vi "Save FITS with Headers coop.vi"(4 "FITS info":T1={"File name"="lsob_demo_0530_LM_20190529_124525_live_C1_00020_001_lev0.0.fits", "Date"="2019-05-29T12:45:25"}, 5 "Camera.lvclass":refnum<class "Camera.lvclass">, 6 "byte order (0:big-endian, network order)":T12(ring), 7 "SCD FITS Cluster":T2={"Wavelength (nm)"=530.15, "Exposure (s)"=0.05, "Tuning Delay (ms)"=1000.0, "Beam Type (-1/1)"=1.0, "Tuning Voltages"=[1.111, 2.222, 3.333, 4.444], "Observer"="observer", "Light Shapping Diffuser"=enum."In Beam", "Comment"="", "Data Type"=enum."HOLE", "Mod Cycles"=0, "SCD Calibration Optics"=enum."1 - Polarizer @0, I+Q", "SCD Emission Line Filter"=enum."1-557.6nm", "Cookbook"="", "COMP-S Calibration Wheel"=enum."Dark", "COMP-S Andover Filter Wheel"=enum."530.3nm/HWB 0.34nm (Fe XIV)", "FOV Rotation (deg)"=66.0, "Objective Lens Position (mm)"=0.0, "Occulter size"=0.0, "Time End"=timestamp(3382374145.421875 s since 1904-01-01), "Acc Exposure (s)"=0.0, "Time Stamp Array"=[], "Camera Serial Number"=[], "Camera Temp"=[], "Camera PI (mm)"=[], "Time Start"=timestamp(3382374145.421875 s since 1904-01-01), "Peripherals"={"ILX controler"=FALSE, "Zone temperatures"=FALSE, "Andor"=FALSE, "Andor 2"=FALSE, "PI Stages"=FALSE, "AISAS mechanisms"=FALSE, "AISAS Mech.lvclass"=refnum, "Zone temp ref"=variant, "FWs"=FALSE}, "FITS paths"=[], "Cameras"=enum."Andor", "load preset cbk"=FALSE, "periodic check count"=0, "COMP-S Calibration Wheel 2"=enum."Dark", "Calib"=enum."Dark", "Abso Aperture"=66.0, "Nominal Aperture"=66.0} {"Nominal Aperture" format="%.1f"; "Abso Aperture" format="%.1f"; "Camera PI (mm)" format="%_3g"; "Acc Exposure (s)" format="%^.3g"; "Occulter size" format="%.2f"; "Objective Lens Position (mm)" min=70.0 max=152.0 format="%.2f"; "FOV Rotation (deg)" format="%.1f"; "Exposure (s)" format="%^.3g"; "Wavelength (nm)" format="%_6g"}, 8 "error in":errorcluster, 9 "Image Data":u32[](array[numeric]), 10 "Image #":i32=1, 11 "FITS File Path":path=path "G:/SCD Data/Level-0/20160930/20160930T203514.fits") -> (0 "error out":errorcluster, 2 "23040 Byte Header":string="SIMPLE  =                              T / CONFORMS TO FITS STANDARD            BITPIX  =                             32 / BITS PER PIXEL                       NAXIS   =                              2 / DATA DIMENSIONS IN FITS FILE         NAXIS1  =                              0 / XDIM (PIXELS)                        NAXIS2  =                              0 / YDIM (PIXELS)                        NAXIS3  =                              4 / 4 POLARIZATION STATES                NAXIS4  =                              1 / 1 CAMERA                             ORIGIN  =                        'AISAS' / SCIENTIFIC GROUP                     OBSERVER=                     'SCHWARTZ' / NAME OF OBSERVER                     TELESCOP=                   '20CM ZEISS' / NAME OF TELESCOPE                    LOCATION=            'LOMNICKY PEAK OBS' / LOCATION OF TELESCOPE                INSTRUME=                          'SCD' / NAME OF INSTRUMENT                   BZERO   =                             0. /  ADU OFFSET                          FOCUS   =                             26 / CAMERA-STAGE POSITION (MM)           ROTPOS  =                           66.0 / ROTATIONAL POSITION (DEG)            DIFFUSER=                      'IN BEAM' / 0=IN BEAM, 1=OUT OF BEAM             FW-WVLNG=                        '557.6' / PRE-FILTER CENTER WAVELENGTH (NM)    FW-CALIB=                         'DARK' / CAL-WHEEL POSITION                   CAM-SN1 =                    'SCC-02209' / CAMERA SERIAL NUMBER                 CAM-TEMP=                       0.000000 / FOCAL PLANE TEMP (C)                 TUNEDLAY=                           1000 / LCVR RELAXATION DELAY (mS)           DATE_OBS=                     '3/7/2011' / DATE OF OBSERVATION START (UTC)      TIME_OBS=                   '212225.421' / TIME OF OBSERVATION (UTC)            EXPOSURE=                       0.050000 / EXPOSURE TIME (S)                    MODC    =                              0 / NUMBER OF IMAGES AT EACH STATE       NLC-1   =                          1.111 / TUNING VOLTAGE-1                     NLC-2   =                          2.222 / TUNING VOLTAGE-2                     NLC-3   =                          3.333 / TUNING VOLTAGE-3                     NLC-4   =                          4.444 / TUNING VOLTAGE-4                     NLC-5   =                          0.000 / TUNING VOLTAGE-5                     BEAM    =                              1 / BEAM (0=ON BAND OR 1=CONTINUUM)      WAVELENG=                         530.15 / WAVELENGTH OF OBS (NM)               COMMHEAD=                             '' / OBSERVER COMMENT                     COOKBOOK=                                / COOKBOOK  LOADED                     COMMENT                                                                         COMMENT                                                                         COMMENT                                                                         COMMENT                                                                         COMMENT                                                                         COMMENT                                                                         COMMENT                                                                         COMMENT                                                                         COMMENT                                                                         COMMENT                                                                         COMMENT                                                                         COMMENT                                                                         COMMENT                                                                         COMMENT                                                                         COMMENT                                                                         COMMENT                                                                         COMMENT                                                                         COMMENT                                                                         COMMENT                                                                         COMMENT                                                                         COMMENT                                                                         COMMENT                                                                         COMMENT                                                                         COMMENT                                                                         COMMENT                                                                         COMMENT                                                                         COMMENT                                                                         COMMENT                                                                         COMMENT                                                                         COMMENT                                                                         COMMENT                                                                         COMMENT                                                                         COMMENT                                                                         COMMENT                                                                         COMMENT                                                                         COMMENT                                                                         COMMENT                                                                         COMMENT                                                                         COMMENT                                                                         COMMENT                                                                         COMMENT                                                                         COMMENT                                                                         COMMENT                                                                         COMMENT                                                                         COMMENT                                                                         COMMENT                                                                         COMMENT                                                                         COMMENT                                                                         COMMENT                                                                         COMMENT                                                                         COMMENT                                                                         COMMENT                                                                         COMMENT                                                                         COMMENT                                                                         COMMENT                                                                         COMMENT                                                                         COMMENT                                                                         COMMENT                                                                         COMMENT                                                                         COMMENT                                                                         COMMENT                                                                         COMMENT                                                                         COMMENT                                                                         COMMENT                                                                         COMMENT                                                                         COMMENT                                                                         COMMENT                                                                         COMMENT                                                                         COMMENT                                                                         COMMENT                                                                         COMMENT                                                                         COMMENT                                                                         COMMENT                                                                         COMMENT                                                                         COMMENT                                                                         COMMENT                                                                         COMMENT                                                                         COMMENT                                                                         COMMENT                                                                         COMMENT                                                                         COMMENT                                                                         COMMENT                                                                         COMMENT                                                                         COMMENT                                                                         COMMENT                                                                         COMMENT                                                                         COMMENT                                                                         COMMENT                                                                         COMMENT                                                                         COMMENT                                                                         COMMENT                                                                         COMMENT                                                                         COMMENT                                                                         COMMENT                                                                         COMMENT                                                                         COMMENT                                                                         COMMENT                                                                         COMMENT                                                                         COMMENT                                                                         COMMENT                                                                         COMMENT                                                                         COMMENT                                                                         COMMENT                                                                         COMMENT                                                                         COMMENT                                                                         COMMENT                                                                         COMMENT                                                                         COMMENT                                                                         COMMENT                                                                         COMMENT                                                                         COMMENT                                                                         COMMENT                                                                         COMMENT                                                                         COMMENT                                                                         COMMENT                                                                         COMMENT                                                                         COMMENT                                                                         COMMENT                                                                         COMMENT                                                                         COMMENT                                                                         COMMENT                                                                         COMMENT                                                                         COMMENT                                                                         COMMENT                                                                         COMMENT                                                                         COMMENT                                                                         COMMENT                                                                         COMMENT                                                                         COMMENT                                                                         COMMENT                                                                         COMMENT                                                                         COMMENT                                                                         COMMENT                                                                         COMMENT                                                                         COMMENT                                                                         COMMENT                                                                         COMMENT                                                                         COMMENT                                                                         COMMENT                                                                         COMMENT                                                                         COMMENT                                                                         COMMENT                                                                         COMMENT                                                                         COMMENT                                                                         COMMENT                                                                         COMMENT                                                                         COMMENT                                                                         COMMENT                                                                         COMMENT                                                                         COMMENT                                                                         COMMENT                                                                         COMMENT                                                                         COMMENT                                                                         COMMENT                                                                         COMMENT                                                                         COMMENT                                                                         COMMENT                                                                         COMMENT                                                                         COMMENT                                                                         COMMENT                                                                         COMMENT                                                                         COMMENT                                                                         COMMENT                                                                         COMMENT                                                                         COMMENT                                                                         COMMENT                                                                         COMMENT                                                                         COMMENT                                                                         COMMENT                                                                         COMMENT                                                                         COMMENT                                                                         COMMENT                                                                         COMMENT                                                                         COMMENT                                                                         COMMENT                                                                         COMMENT                                                                         COMMENT                                                                         COMMENT                                                                         COMMENT                                                                         COMMENT                                                                         COMMENT                                                                         COMMENT                                                                         COMMENT                                                                         COMMENT                                                                         COMMENT                                                                         COMMENT                                                                         COMMENT                                                                         COMMENT                                                                         COMMENT                                                                         COMMENT                                                                         COMMENT                                                                         COMMENT                                                                         COMMENT                                                                         COMMENT                                                                         COMMENT                                                                         COMMENT                                                                         COMMENT                                                                         COMMENT                                                                         COMMENT                                                                         COMMENT                                                                         COMMENT                                                                         COMMENT                                                                         COMMENT                                                                         COMMENT                                                                         COMMENT                                                                         COMMENT                                                                         COMMENT                                                                         COMMENT                                                                         COMMENT                                                                         COMMENT                                                                         COMMENT                                                                         COMMENT                                                                         COMMENT                                                                         COMMENT                                                                         COMMENT                                                                         COMMENT                                                                         COMMENT                                                                         COMMENT                                                                         COMMENT                                                                         COMMENT                                                                         COMMENT                                                                         COMMENT                                                                         COMMENT                                                                         COMMENT                                                                         COMMENT                                                                         COMMENT                                                                         COMMENT                                                                         COMMENT                                                                         COMMENT                                                                         COMMENT                                                                         COMMENT                                                                         COMMENT                                                                         COMMENT                                                                         COMMENT                                                                         COMMENT                                                                         COMMENT                                                                         COMMENT                                                                         COMMENT                                                                         COMMENT                                                                         COMMENT                                                                         COMMENT                                                                         COMMENT                                                                         COMMENT                                                                         COMMENT                                                                         COMMENT                                                                         COMMENT                                                                         COMMENT                                                                         COMMENT                                                                         COMMENT                                                                         COMMENT                                                                         COMMENT                                                                         COMMENT                                                                         COMMENT                                                                         END                                                                             ", 3 "FITS Path Out":path=path "G:/SCD Data/Level-0/20160930/20160930T203514.fits")   [LabVIEW 2014]
doc: "Duplicate first measurement\nand put it in first element of\nmeasurement array. This\nis a dummy measurement for the\nprimary header. This is because\nwe don't want any images associated\nwith the primary HDU, just the \nextensions. In the Make FITS\nHeaders VI, the NAXIS is set to 0 in\nthis primary HDU"
uses:
  Controls/SCD - FITS Cluster.ctl
  AISAS/Mech/AISAS Mech.lvclass
  AISAS/Controls/Diffuser.ctl
  Controls/FITS Data type.ctl
  Controls/SCD - Calibration Optics Filter Wheel.ctl
  Controls/SCD - EDT - Emission Line Filter Wheel.ctl
  Controls/CoMP-S Controls/Polarization Optics Filter Wheel.ctl
  Controls/CoMP-S Controls/Emission Line Filter Wheel.ctl
  AISAS/Controls/focus.ctl
  Controls/peripherals.ctl
  Controls/Cameras select.ctl
  Controls/Fits info.ctl
  Camera/Camera/Camera.lvclass
  Controls/Globals.vi
panel:
  out "NAXIS":string
  out "# Images in Vector":i32=4
  out "Length of Vector":i32=22118400
  out "Total Pixels":i64=5529600
  out "AOI Height":i64=2160
  out "AOI Width":i64=2560
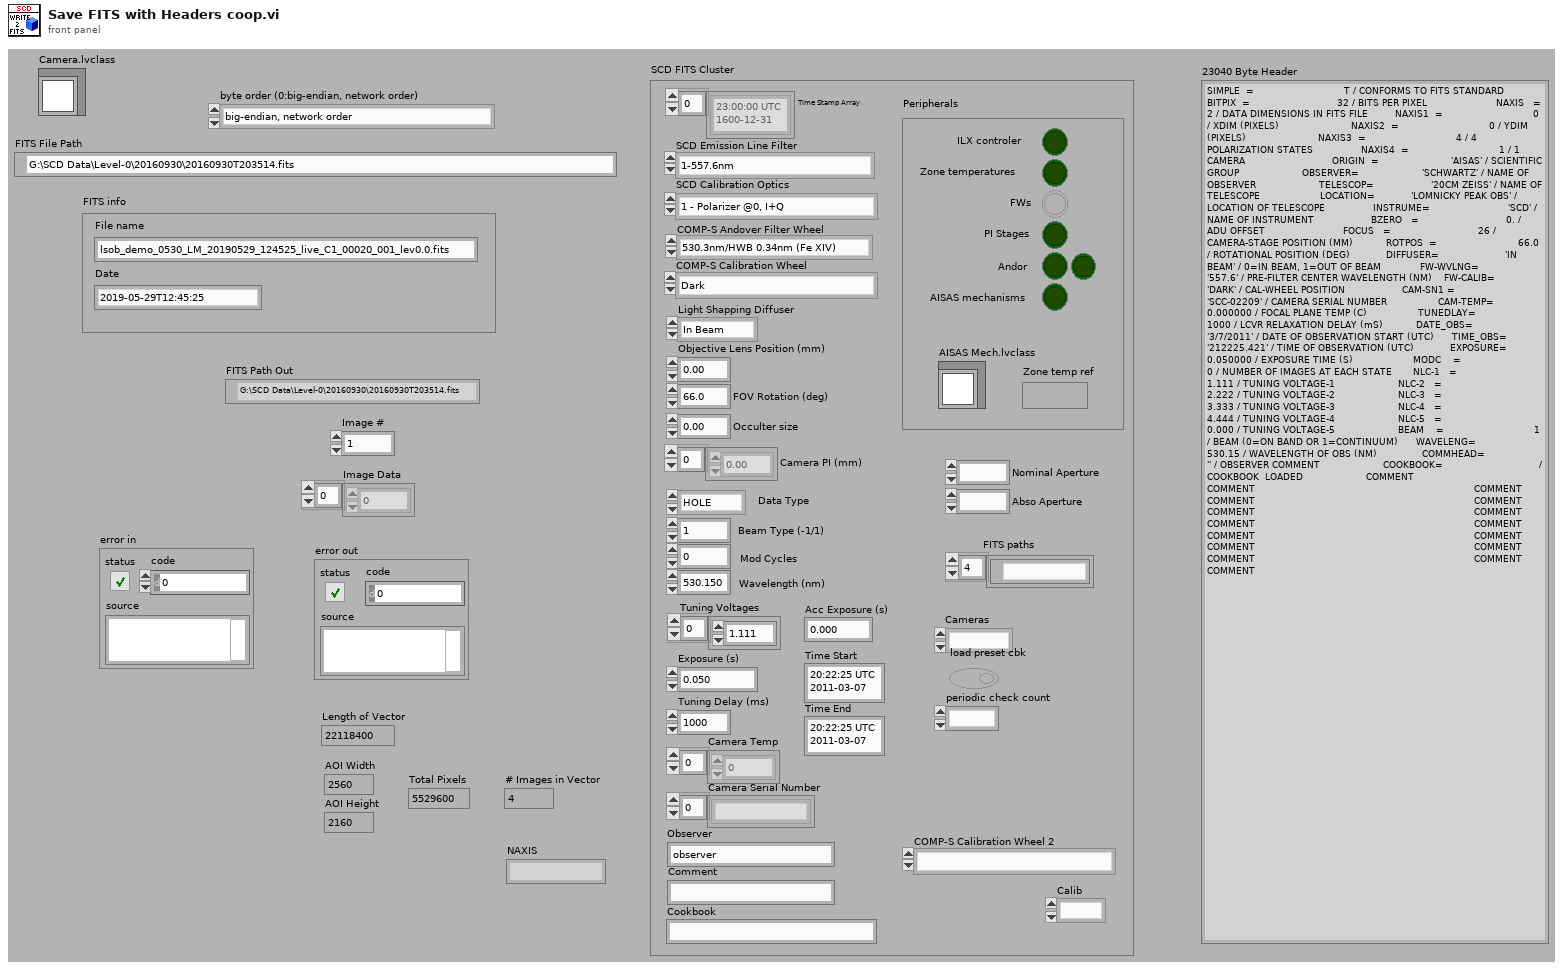
[diagram p1: front panel]
types:
  T1 = typedef "Fits info.ctl" = cluster{"File name":string, "Date":string}
  T2 = typedef "SCD - FITS Cluster.ctl" = cluster{"Wavelength (nm)":dbl, "Exposure (s)":dbl, "Tuning Delay (ms)":dbl, "Beam Type (-1/1)":dbl, "Tuning Voltages":dbl[], "Observer":string, "Light Shapping Diffuser":T3, "Comment":string, "Data Type":T4, "Mod Cycles":u16, "SCD Calibration Optics":T5, "SCD Emission Line Filter":T6, "Cookbook":string, "COMP-S Calibration Wheel":T7, "COMP-S Andover Filter Wheel":T8, "FOV Rotation (deg)":dbl, "Objective Lens Position (mm)":T9, "Occulter size":dbl, "Time End":timestamp, "Acc Exposure (s)":dbl, "Time Stamp Array":timestamp[], "Camera Serial Number":string[], "Camera Temp":dbl[], "Camera PI (mm)":dbl[], "Time Start":timestamp, "Peripherals":T10, "FITS paths":path[], "Cameras":T11, "load preset cbk":bool, "periodic check count":i32, "COMP-S Calibration Wheel 2":T7, "Calib":enum16{"Dark", "Flat"}, "Abso Aperture":dbl, "Nominal Aperture":dbl}
  T3 = typedef "Diffuser.ctl" = enum16{"Out of Beam", "In Beam"}
  T4 = typedef "FITS Data type.ctl" = enum16{"LIVE", "DARK", "FLAT", "CALI", "OBSE", "ABSO", "AURE", "TARG", "OBJE", "HOLE", "OREX", "THRO", "CHIP"}
  T5 = typedef "SCD - Calibration Optics Filter Wheel.ctl" = enum16{"1 - Polarizer @0, I+Q", "2 - Polarizer @90, I-Q", "3 - Polarizer @45, I+U", "4 - Polarizer @135, I-U", "5 - Polarizer @0, Retarder @45, I+V", "6 - Polarizer @0, Retarder @135, I-V", "7 - Dark", "8 - Clear", "9 - N/A"}
  T6 = typedef "SCD - EDT - Emission Line Filter Wheel.ctl" = enum16{"1-557.6nm", "2-587.6nm", "3-589.6nm", "4-630.2nm", "5-656.4nm", "6-849.8nm", "7-854.2nm", "8-866.2nm", "9-1083.0nm"}
  T7 = typedef "Polarization Optics Filter Wheel.ctl" = enum16{"Dark", "Clear", "Exchange Lens", "Polarizer @0, I+Q", "Polarizer @90, I-Q", "Polarizer @45, I+U", "Polarizer @135, I-U", "Polarizer @0, Retarder @45, I+V", "Polarizer @0, Retarder @135, I-V"}
  T8 = typedef "Emission Line Filter Wheel.ctl" = enum16{"530.3nm/HWB 0.34nm (Fe XIV)", "587.6nm/HBW 0.44nm (He I D3)", "637.5nm/HBW 0.53nm (Fe X)", "656.3nm/HBW 0.57nm (H-Alpha)", "789.2nm/HBW 0.85nm (Fe XI)", "854.2nm/HBW 1.01nm (Ca I)", "1074.7nm/HBW 2.34nm (Fe XIII)", "1079.8nm/HBW 1.64nm (Fe XIII)", "1083.0nm/HBW 1.66nm (He I)"}
  T9 = typedef "focus.ctl" = dbl
  T10 = typedef "peripherals.ctl" = cluster{"ILX controler":bool, "Zone temperatures":bool, "Andor":bool, "Andor 2":bool, "PI Stages":bool, "AISAS mechanisms":bool, "AISAS Mech.lvclass":refnum<class "AISAS Mech.lvclass">, "Zone temp ref":variant, "FWs":bool}
  T11 = typedef "Cameras select.ctl" = enum16{"Andor", "GDR"}
  T12 = enum16{"big-endian, network order", "native, host order", "little-endian"}
  T13 = enum16{"open", "replace", "create", "open or create", "replace or create", "replace or create with confirmation"}
  T14 = typedef "beaning.ctl" = enum16{"1x1", "2x2", "3x3", "4x4", "8x8"}
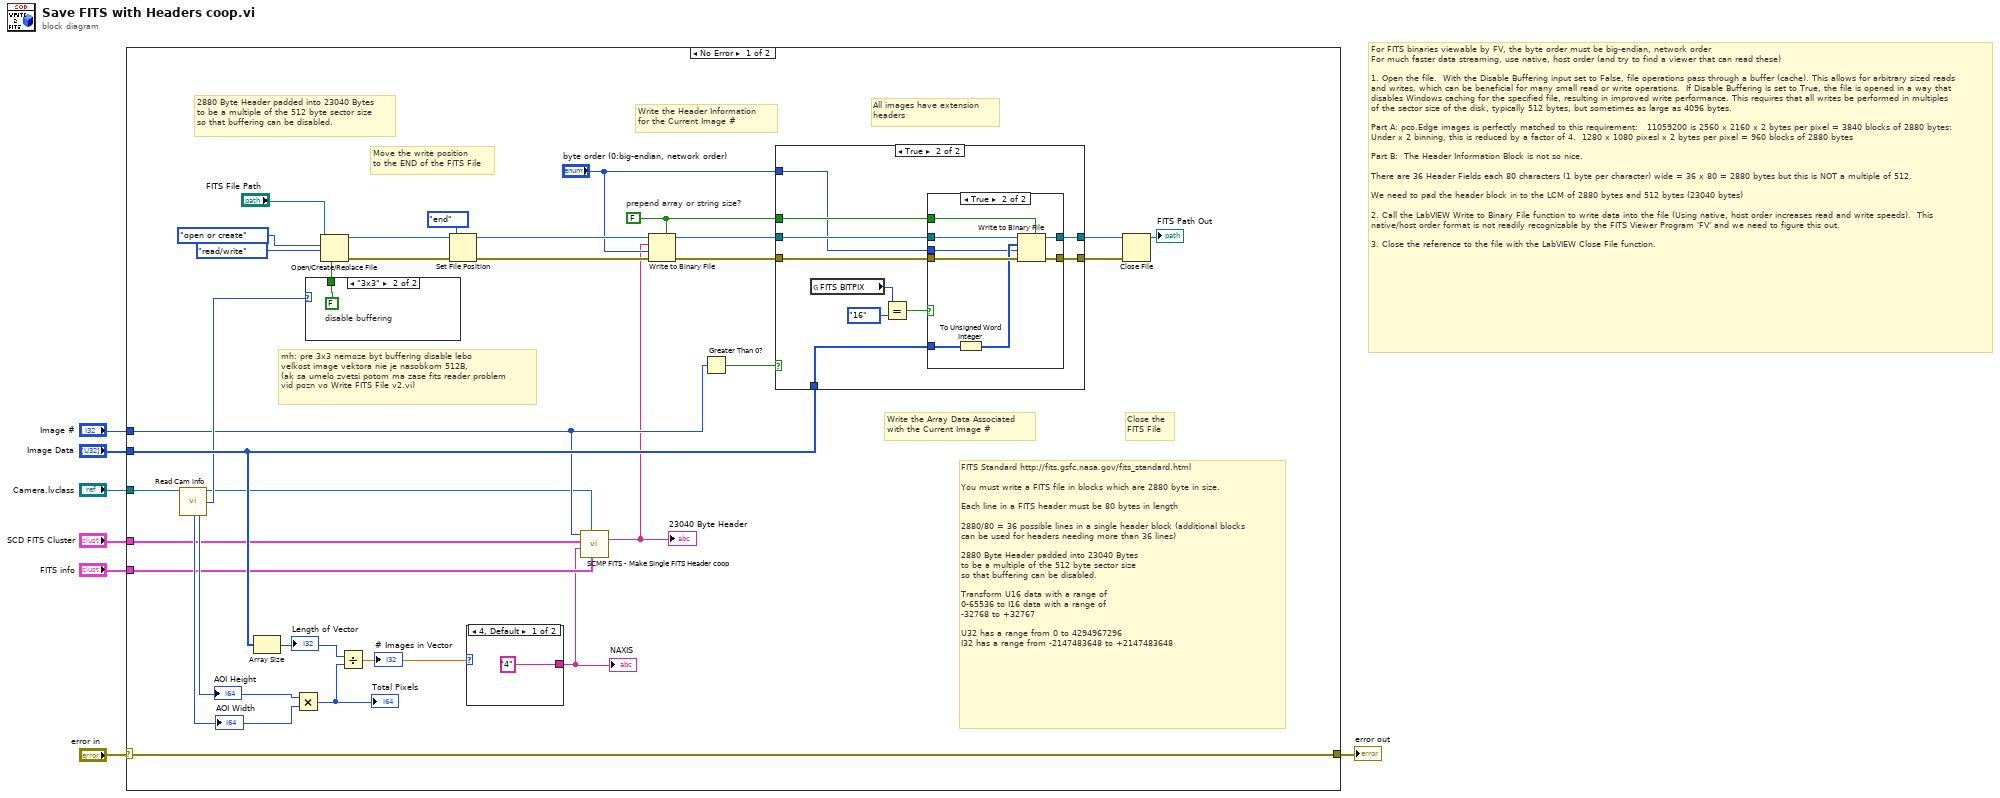
[diagram p0: block diagram]
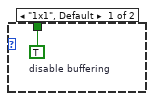
[diagram p2: hidden frame]
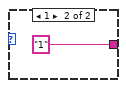
[diagram p3: hidden frame]
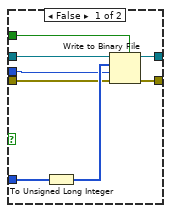
[diagram p5: hidden frame]
diagram:
  # "For FITS binaries viewable by FV, the byte order must be big-endian, network order\nFor much faster data streaming, use native, host order (and try to find a viewer that can read these)\n\n1. Open the file.  With the Disable Buffering input set to False, file operations pass through a buffer (cache). This allows for arbitrary sized reads and writes, which can be beneficial for many small read or write operations.  If Disable Buffering is set to True, the file is opened in a way that disables Windows caching for the specified file, resulting in improved write performance. This requires that all writes be performed in multiples of the sector size of the disk, typically 512 bytes, but sometimes as large as 4096 bytes.\n\nPart A: pco.Edge images is perfectly matched to this requirement:   11059200 is 2560 x 2160 x 2 bytes per pixel = 3840 blocks of 2880 bytes:  Under x 2 binning, this is reduced by a factor of 4.  1280 x 1080 pixesl x 2 bytes per pixel = 960 blocks of 2880 bytes\n\nPart B:  The Header Information Block is not so nice.  \n\nThere are 36 Header Fields each 80 characters (1 byte per character) wide = 36 x 80 = 2880 bytes but this is NOT a multiple of 512.\n\nWe need to pad the header block in to the LCM of 2880 bytes and 512 bytes (23040 bytes)\n\n2. Call the LabVIEW Write to Binary File function to write data into the file (Using native, host order increases read and write speeds).  This native/host order format is not readily recognizable by the FITS Viewer Program 'FV' and we need to figure this out.\n\n3. Close the reference to the file with the LabVIEW Close File function."
  n1 = case shown="No Error" "error in" {
    selector: "error in" -> [w33 w72]
    tunnel: [w33 w72] -> w6
    tunnel: "Image #" -> [w13 _]
    tunnel: "Image Data" -> [w18 _]
    tunnel: "SCD FITS Cluster" -> [w12 _]
    tunnel: "FITS info" -> [w11 _]
    tunnel: "Camera.lvclass" -> [w14 _]
    frame No Error {
      w30 = FALSE  # prepend array or string size?
      # "mh: pre 3x3 nemoze byt buffering disable lebo\nvelkost image vektora nie je nasobkom 512B,\n(ak sa umelo zvetsi potom ma zase fits reader problem\nvid pozn vo Write FITS File v2.vi)"
      # "All images have extension \nheaders"
      # "2880 Byte Header padded into 23040 Bytes\nto be a multiple of the 512 byte sector size\nso that buffering can be disabled."
      # "FITS Standard http://fits.gsfc.nasa.gov/fits_standard.html\n\nYou must write a FITS file in blocks which are 2880 byte in size.\n\nEach line in a FITS header must be 80 bytes in length\n\n2880/80 = 36 possible lines in a single header block (additional blocks\ncan be used for headers needing more than 36 lines)\n\n2880 Byte Header padded into 23040 Bytes\nto be a multiple of the 512 byte sector size\nso that buffering can be disabled.\n\nTransform U16 data with a range of\n0-65536 to I16 data with a range of\n-32768 to +32767\n\nU32 has a range from 0 to 4294967296\nI32 has a range from -2147483648 to +2147483648"
      # "Close the \nFITS File"
      # "Write the Array Data Associated\nwith the Current Image #"
      # "Write the Header Information\nfor the Current Image #"
      # "Move the write position\nto the END of the FITS File"
      n2 = call-dynamic "Read Cam info.vi"("Camera in"=w14) -> ("Camera out"=w8:refnum<class "Camera.lvclass">, "Binning"=w17:T14, "AOI Width"=w15:i32, "AOI Height"=w16:i32)  [unwired: 5 in, 6 out]
      "AOI Width" <- w15
      "AOI Height" <- w16
      n3 = Array Size(array=w18) -> (size(s)=w23:i32)
      "Length of Vector" <- w23
      n4 = Multiply(x=w16, y=w15) -> (x*y=w22:i32)
      "Total Pixels" <- w22
      n5 = case shown="\"3x3\"" w17 {
        tunnel: [w40 w41] -> w34
        frame "1x1", Default {
          w40 = TRUE  # disable buffering
        }
        frame "3x3" {
          w41 = FALSE  # disable buffering
        }
      }
      n6 = Open/Create/Replace File(file path (use dialog)="FITS File Path", operation (0:open)=T13."open or create", access (0:read/write)=enum16{"read/write", "read-only", "write-only"}."read/write", disable buffering (F)=w34) -> (refnum out=w26:refnum<file>, error out=w27:errorcluster)  [unwired: 1 in, 2 out]
      n7 = Divide(x=w23, y=w22) -> (x/y=w21:dbl)
      "# Images in Vector" <- w21
      n8 = Set File Position(refnum=w26, from (0:start)=enum16{"start", "end", "current"}."end" ("pos mode (0:2)"), error in=w27) -> (refnum out=w25:refnum<file>, error out=w24:errorcluster)  [unwired: 1 out]
      n9 = case shown="4, Default" w21 {
        tunnel: ["4" ("NAXIS") "1" ("NAXIS")] -> w9
        frame 4, Default {
        }
        frame 1 {
        }
      }
      "NAXIS" <- w9
      n10 = call "SCMP FITS - Make Single FITS Header coop.vi"("FITS info"=w11, "Camera.lvclass"=w8, "NAXIS"=w9, "FITS Header"=w12, "Image #"=w13) -> ("23040 Byte Header"=w10:string)  [unwired: 4 in, 2 out]
      "23040 Byte Header" <- w10
      n11 = Write to Binary File(file (use dialog)=w25, data=w10, error in=w24, 5:w30, 9:"byte order (0:big-endian, network order)") -> (refnum out=w31:refnum<file>, error out=w32:errorcluster)  [unwired: 2 out]
      n12 = Greater Than 0?(x=w13) -> (x > 0?=w29:bool)
      n13 = case shown="True" w29 {
        tunnel: [w44 w55] -> w39
        tunnel: [w45 w54] -> w38
        tunnel: w32 -> [w44 w51]
        tunnel: w31 -> [w45 w52]
        tunnel: w30 -> [_ w53]
        tunnel: w18 -> [_ w50]
        tunnel: "byte order (0:big-endian, network order)" -> [_ w46]
        frame False {
          # "Primary Headers have no associated image.  \nAll we've done so far is to create a blank FITS \nfile and write a Primary Header"
        }
        frame True {
          n14 = global read "Globals.vi" "FITS BITPIX"() -> (w48:enum16{"16", "32"})
          n15 = Equal?(x=w48, y=enum16{"16", "32"}."16") -> (x = y?=w47:bool)
          n16 = case shown="True" w47 {
            tunnel: [w57 w71] -> w55
            tunnel: [w56 w70] -> w54
            tunnel: w53 -> [w60 w69]
            tunnel: w52 -> [w61 w68]
            tunnel: w51 -> [w62 w67]
            tunnel: w50 -> [w59 w66]
            tunnel: w46 -> [w58 w64]
            frame False {
              n17 = To Unsigned Long Integer(number=w59) -> (unsigned 32bit integer=w63:u32[])
              n18 = Write to Binary File(file (use dialog)=w61, data=w63, error in=w62, 5:w60, 9:w58) -> (refnum out=w56:refnum<file>, error out=w57:errorcluster)  [unwired: 2 out]
            }
            frame True {
              n19 = To Unsigned Word Integer(number=w66) -> (unsigned 16bit integer=w65:u16[])
              n20 = Write to Binary File(file (use dialog)=w68, data=w65, error in=w67, 5:w69, 9:w64) -> (refnum out=w70:refnum<file>, error out=w71:errorcluster)  [unwired: 2 out]
            }
          }
        }
      }
      n21 = Close File(refnum=w38, error in=w39) -> (path=→"FITS Path Out":path)  [unwired: 1 out]
    }
    frame Error {
    }
  }
  "error out" <- w6
